vi "GUI - HDF (V1.00).vi"(0 "Time Data IN":refnum<class "GSwFormDSP.lvclass">, 5 "error in (no error)":errorcluster, 7 "Application Name":string="GSwForm", 9 "State Queue":string[](array[string])=["SC: Initialize"], 11 "HDF - READ":path, 13 "HDF - WRITE":path) -> (14 "Time Data DUP":refnum<class "GSwFormDSP.lvclass">, 19 "error out":errorcluster)   [LabVIEW 2020, in "HeadAcousticHDF.lvclass"]
uses:
  HeadAcousticHDF.lvclass
  API/GSwFormDSP_class/GSwFormDSP.lvclass
  <vilib>/Utility/sysdir.llb/System Directory Type.ctl
  C:/Users/fcharett/docsWork/coding/20openSourceSPWB/API/Generic Utilities_class/Generic Utilities.lvclass
  <vilib>/addons/_AddQ/G#Object/G#Object.lvclass
  API/Generic Utilities_class/Generic Utilities.lvclass
panel:
  in  "Task":enum32{"IO File", "File Info", "Settings"}(tab)
  out "Time Data":waveform(dbl)[](graph)
  in  "READ - Select HDF File":bool
  in  "WRITE - Select Wave File":bool
  in  "Select Channel":u16(ring)
  in  "File Info":bool
  out "State History":string[](array[string])
  out "State Index":i32
  in  "Exit":bool
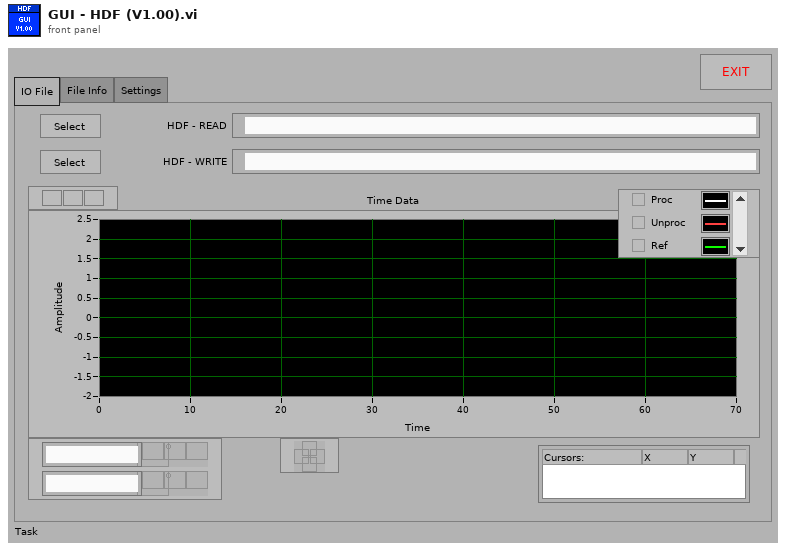
[diagram p1: front panel]
types:
  T1 = enum32{"Invalid", "Standard", "Closed", "Hidden", "Minimized", "Maximized"}
  T2 = typedef "System Directory Type.ctl" = i32
  T3 = cluster{"Name":string, "Unit":string, "Duration (sec)":dbl}[][]
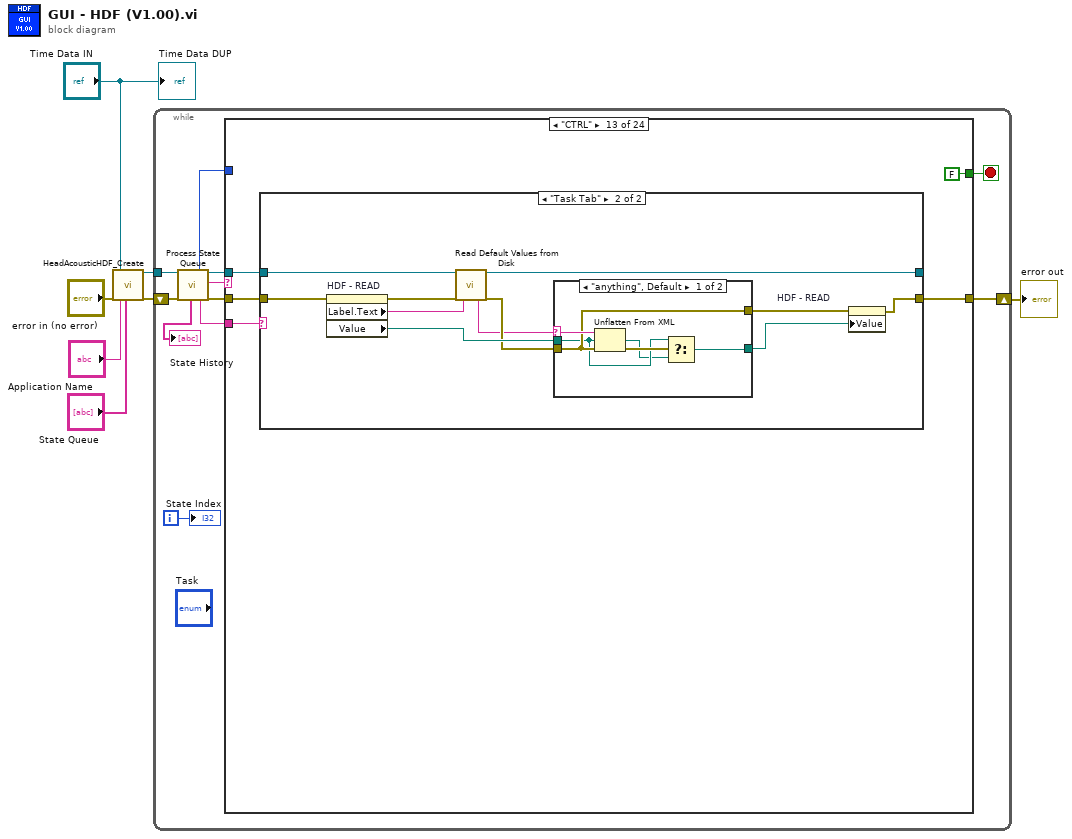
[diagram p0: block diagram]
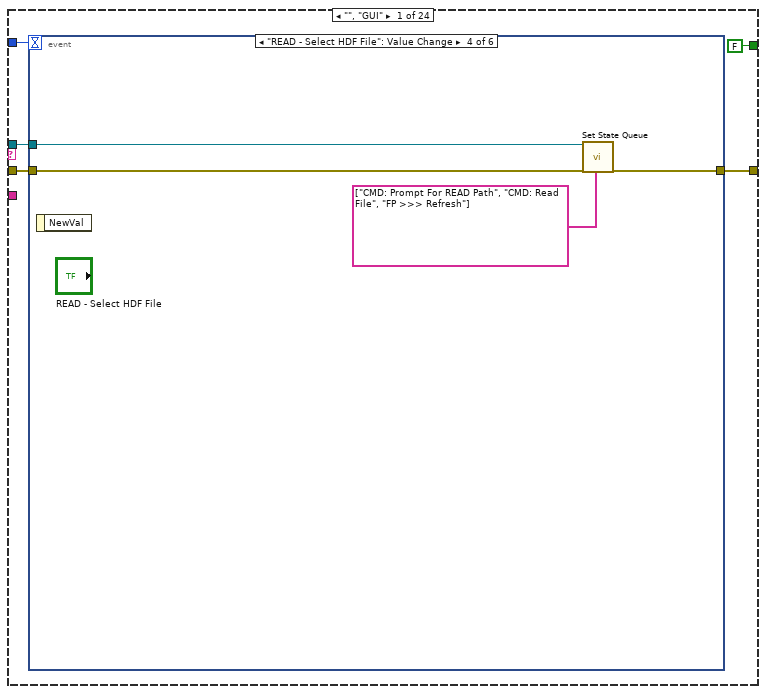
[diagram p2: hidden frame]
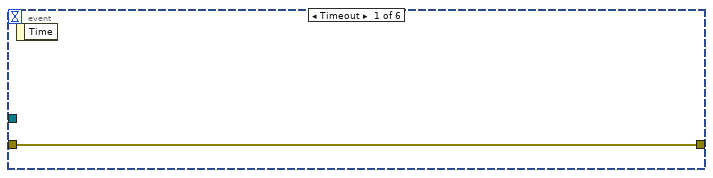
[diagram p3: hidden frame]
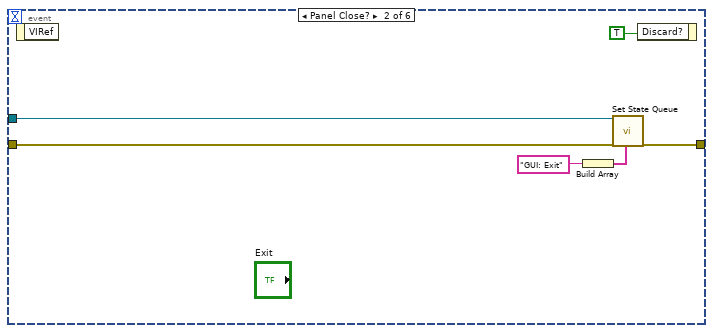
[diagram p4: hidden frame]
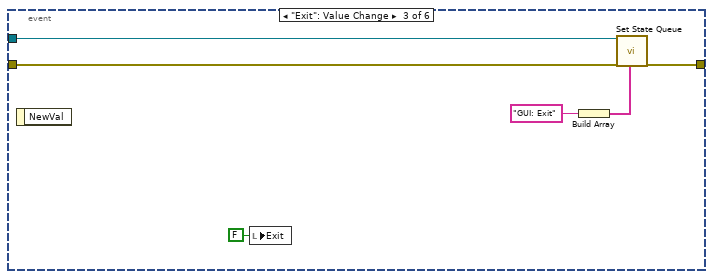
[diagram p5: hidden frame]
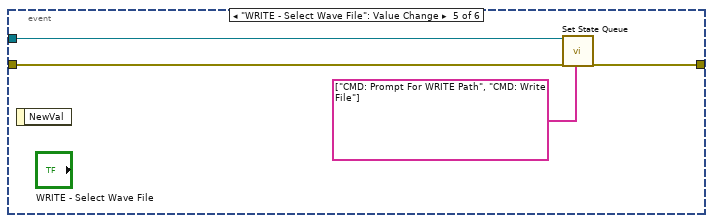
[diagram p6: hidden frame]
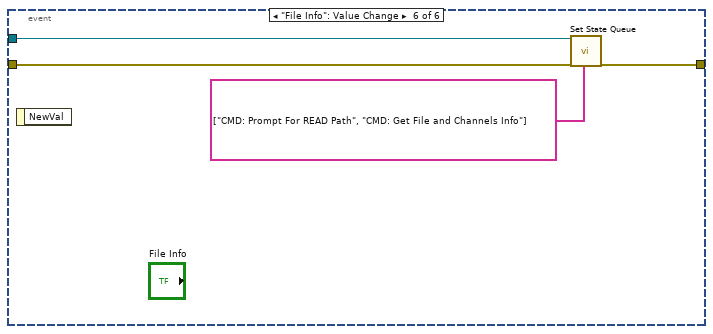
[diagram p7: hidden frame]
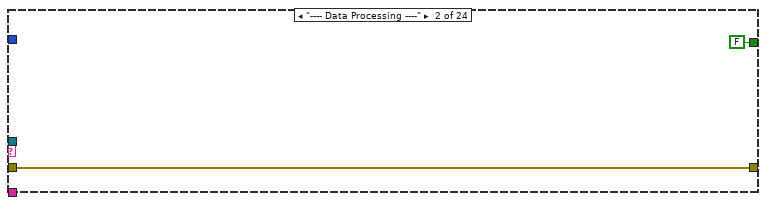
[diagram p8: hidden frame]
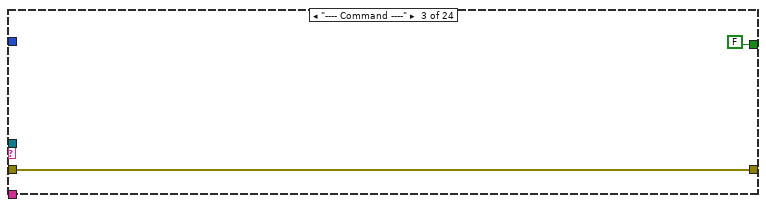
[diagram p9: hidden frame]
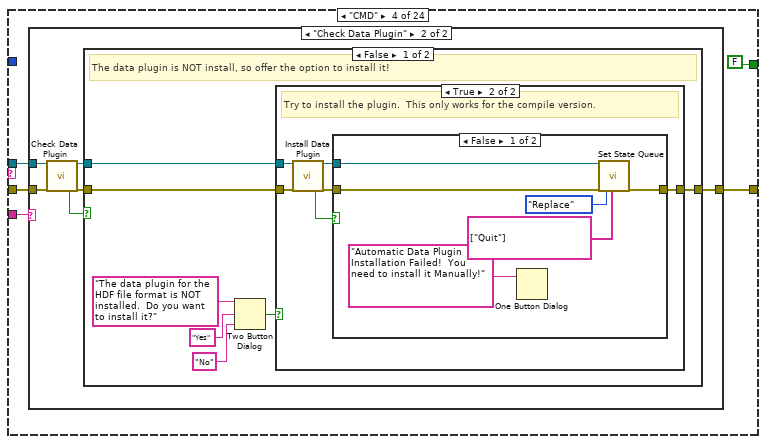
[diagram p10: hidden frame]
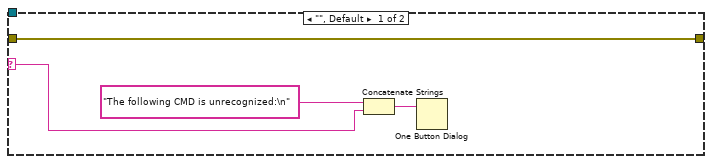
[diagram p11: hidden frame]
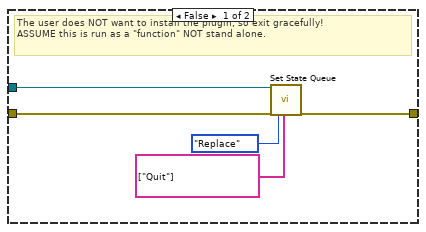
[diagram p12: hidden frame]
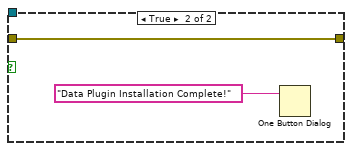
[diagram p13: hidden frame]
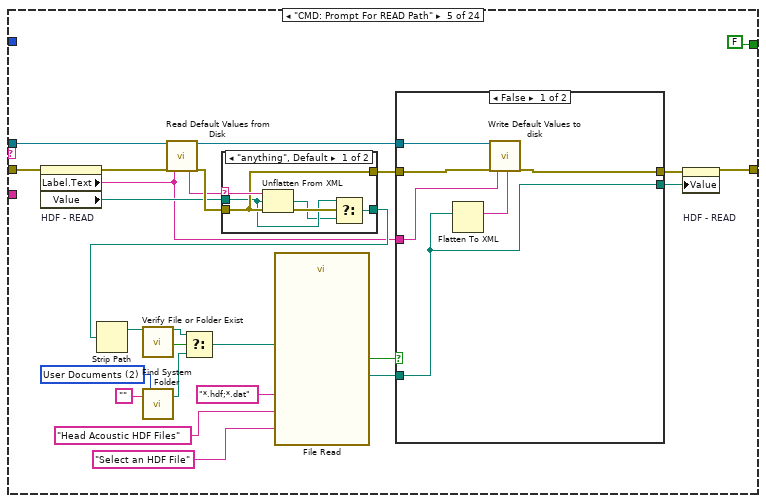
[diagram p15: hidden frame]
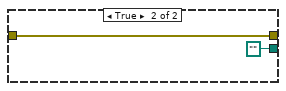
[diagram p16: hidden frame]
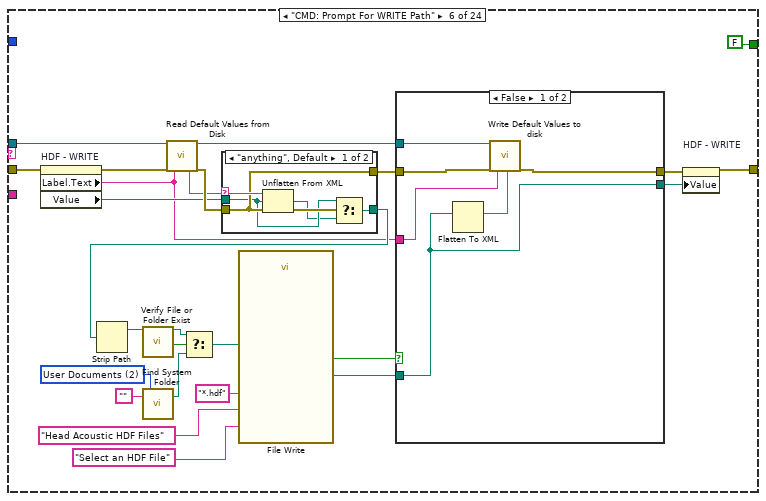
[diagram p18: hidden frame]
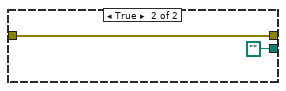
[diagram p19: hidden frame]
diagram:
  n1 = call "HeadAcousticHDF_Create.vi"("error in (no error)"="error in (no error)", "Time Data"="Time Data IN", "Application Name"="Application Name", "State Queue"="State Queue") -> ("reference out"=w7:refnum<class "HeadAcousticHDF.lvclass">, "error out"=w6:errorcluster)  [unwired: 14 in]
  n2 = while {
    shift-right: [w9] -> w2
    shift-left: w6 -> [w15]
    tunnel: w7 -> [w16]
    i -> [w17]
    stop <- w18 stop-if-true
    n3 = call "Process State Queue.vi"("reference in"=w16, "error in (no error)"=w15) -> ("State History"=→"State History":string[], "Timeout"=w14:i32, "State Option"=w11:string, "reference out"=w13:refnum<class "HeadAcousticHDF.lvclass">, "Current State"=w12:string, "error out"=w10:errorcluster)  [unwired: 10 in, 2 out]
    n4 = case shown="\"CTRL\"" w12 {
      selector: w12 -> [_ _ _ _ _ _ _ _ _ _ _ _ _ _ _ _ _ _ _ _ w403 _ _ _]
      tunnel: w13 -> [w21 _ _ w53 w119 w161 w183 w195 w208 _ w231 _ w237 w267 _ w308 w327 w360 w385 _ _ _ _ w411]
      tunnel: [FALSE FALSE FALSE FALSE FALSE FALSE FALSE FALSE FALSE FALSE FALSE FALSE FALSE FALSE FALSE FALSE TRUE FALSE FALSE FALSE FALSE FALSE FALSE TRUE] -> w18
      tunnel: w14 -> [w22 _ _ _ _ _ _ _ _ _ _ _ _ _ _ _ _ _ _ _ _ _ _ _]
      tunnel: w11 -> [_ _ _ w56 _ _ _ _ _ _ _ _ w238 w264 _ _ _ w369 _ _ _ _ _ _]
      tunnel: w10 -> [w20 w49 w51 w54 w118 w160 w182 w194 w209 w226 w230 w233 w235 w266 w293 w305 w324 w359 w386 w399 w401 w406 w409 w412]
      tunnel: [w19 w49 w51 w55 w102 w146 w181 w193 w204 w226 w229 w233 w236 w265 w293 w295 w323 w357 w382 w399 w401 errorcluster {"status"=FALSE, "code"=0, "source"=""} ("error out") w409 w413] -> w9
      frame "", "GUI" {
        n5 = event shown="[3] \"READ - Select HDF File\": Value Change" {
          selector: _ -> [_ _ _ _ _ _]
          dyn-events: _ -> [_ _ _ _ _ _]
          timeout: w22 -> [_ _ _ _ _ _]
          tunnel: w21 -> [_ w28 w34 w39 w43 w45]
          tunnel: w20 -> [w24 w27 w32 w38 w42 w46]
          tunnel: [w24 w26 w33 w40 w44 w47] -> w19
          event Timeout {
            n6 = event-data() -> ()  [unwired: 1 in, 1 out]
          }
          event Panel Close? {
            n7 = event-data() -> ()  [unwired: 1 in, 1 out]
            n8 = Build Array("GUI: Exit") -> (w25:string[])
            n9 = call "Set State Queue.vi"("reference in"=w28, "error in (no error)"=w27, "State Queue"=w25) -> ("error out"=w26:errorcluster)  [unwired: 15 in, 1 out]
            n10 = event-data("Discard?"=TRUE) -> ()  [unwired: 1 in, 1 out]
          }
          event "Exit": Value Change {
            n11 = event-data() -> ()  [unwired: 1 in, 1 out]
            n12 = local write "Exit"(FALSE ("Exit")) -> ()
            n13 = Build Array("GUI: Exit") -> (w31:string[])
            n14 = call "Set State Queue.vi"("reference in"=w34, "error in (no error)"=w32, "State Queue"=w31) -> ("error out"=w33:errorcluster)  [unwired: 15 in, 1 out]
          }
          event "READ - Select HDF File": Value Change {
            n15 = event-data() -> ()  [unwired: 1 in, 1 out]
            n16 = call "Set State Queue.vi"("reference in"=w39, "error in (no error)"=w38, "State Queue"=string[] ["CMD: Prompt For READ Path", "CMD: Read File", "FP >>> Refresh"]) -> ("error out"=w40:errorcluster)  [unwired: 15 in, 1 out]
          }
          event "WRITE - Select Wave File": Value Change {
            n17 = event-data() -> ()  [unwired: 1 in, 1 out]
            n18 = call "Set State Queue.vi"("reference in"=w43, "error in (no error)"=w42, "State Queue"=string[] ["CMD: Prompt For WRITE Path", "CMD: Write File"]) -> ("error out"=w44:errorcluster)  [unwired: 15 in, 1 out]
          }
          event "File Info": Value Change {
            n19 = event-data() -> ()  [unwired: 1 in, 1 out]
            n20 = call "Set State Queue.vi"("reference in"=w45, "error in (no error)"=w46, "State Queue"=string[] ["CMD: Prompt For READ Path", "CMD: Get File and Channels Info"]) -> ("error out"=w47:errorcluster)  [unwired: 15 in, 1 out]
          }
        }
      }
      frame "---- Data Processing ----" {
      }
      frame "---- Command ----" {
      }
      frame "CMD" {
        n21 = case shown="\"Check Data Plugin\"" w56 {
          selector: w56 -> [w59 _]
          tunnel: [w58 w64] -> w55
          tunnel: w54 -> [w58 w66]
          tunnel: w53 -> [_ w67]
          frame "", Default {
            n22 = Concatenate Strings("The following CMD is unrecognized:\n", w59) -> (w60:string)
            n23 = One Button Dialog(message=w60) -> ()  [unwired: 1 in, 1 out]
          }
          frame "Check Data Plugin" {
            n24 = call "Check Data Plugin.vi"("reference in"=w67, "error in (no error)"=w66) -> ("HDF Plugin OK?"=w65:bool, "reference out"=w62:refnum<class "HeadAcousticHDF.lvclass">, "error out"=w63:errorcluster)  [unwired: 15 in]
            n25 = case shown="False" w65 {
              tunnel: [w69 w94] -> w64
              tunnel: w63 -> [w70 w94]
              tunnel: w62 -> [w71 _]
              frame False {
                # "The data plugin is NOT install, so offer the option to install it!"
                n26 = Two Button Dialog(message="The data plugin for the HDF file format is NOT installed.  Do you want to install it?", 1:"No" ("F button name (\"Cancel\")"), 2:"Yes" ("T button name (\"OK\")")) -> (T button?=w72:bool)
                n27 = case shown="True" w72 {
                  tunnel: w71 -> [w79 w85]
                  tunnel: w70 -> [w78 w84]
                  tunnel: [w77 w82] -> w69
                  frame False {
                    # "The user does NOT want to install the plugin, so exit gracefully!\nASSUME this is run as a \"function\" NOT stand alone."
                    n28 = call "Set State Queue.vi"("reference in"=w79, "error in (no error)"=w78, "State Queue Options"=enum16{"Replace", "Append", "Prepend"}."Replace", "State Queue"=string[] ["Quit"]) -> ("error out"=w77:errorcluster)  [unwired: 14 in, 1 out]
                  }
                  frame True {
                    # "Try to install the plugin.  This only works for the compile version."
                    n29 = call "Install Data Plugin.vi"("reference in"=w85, "error in (no error)"=w84) -> ("Successful Install?"=w83:bool, "reference out"=w80:refnum<class "HeadAcousticHDF.lvclass">, "error out"=w81:errorcluster)  [unwired: 15 in]
                    n30 = case shown="False" w83 {
                      tunnel: [w86 w92] -> w82
                      tunnel: w81 -> [w87 w92]
                      tunnel: w80 -> [w88 _]
                      frame False {
                        n31 = One Button Dialog(message="Automatic Data Plugin Installation Failed!  You need to install it Manually!") -> ()  [unwired: 1 in, 1 out]
                        n32 = call "Set State Queue.vi"("reference in"=w88, "error in (no error)"=w87, "State Queue Options"=enum16{"Replace", "Append", "Prepend"}."Replace", "State Queue"=string[] ["Quit"]) -> ("error out"=w86:errorcluster)  [unwired: 14 in, 1 out]
                      }
                      frame True {
                        n33 = One Button Dialog(message="Data Plugin Installation Complete!") -> ()  [unwired: 1 in, 1 out]
                      }
                    }
                  }
                }
              }
              frame True {
                # "The data plugin is OK"
              }
            }
          }
        }
      }
      frame "CMD: Prompt For READ Path" {
        w109 = T2 2 items=["User Home"=0, "User Desktop"=1, "User Documents"=2, "User Application Data"=3, "User Preferences"=4, "User Temporary"=5, "Public Documents"=6, "Public Application Data"=7, "Public Preferences"=8, "Public Cache"=13, "System Core Libraries"=9, "System Installed Libraries"=10, "Application Files"=11, "Boot Volume Root"=12] ("system directory type")
        n34 = property on="HDF - READ" class="Path"(error in=w118) -> (error out=w117:errorcluster, "Label.Text"=w97:string, "Value"=w115:path)  [unwired: 1 in, 1 out]
        n35 = call "Find System Folder.vi"("Application Name"="", "system directory type"=w109) -> ("System Folder"=w108:path)  [unwired: 16 in, 1 out]
        n36 = call-dynamic "Read Default Values from Disk.vi"("reference in"=w119, "error in (no error)"=w117, "Control Label"=w97) -> ("Value (XML String)"=w95:string, "reference out"=w98:refnum<class "HeadAcousticHDF.lvclass">, "error out"=w116:errorcluster)  [unwired: 14 in]
        n37 = case shown="\"anything\", Default" w95 {
          selector: w95 -> [w134 _]
          tunnel: [w129 w136] -> w114
          tunnel: w115 -> [w131 w136]
          tunnel: w116 -> [w132 w135]
          tunnel: [w132 w135] -> w100
          frame "anything", Default {
            n38 = Unflatten From XML(xml string=w134, type=w131, error in (no error)=w132) -> (value=w130:path, error out=w133:errorcluster)
            n39 = Select(t=w131, s=w133, f=w130) -> (s? t:f=w129:path)
          }
          frame "" {
            # "Either the file was not found or there was some error"
          }
        }
        n40 = Strip Path(path=w114) -> (stripped path=w113:path)  [unwired: 1 out]
        n41 = call "Verify File or Folder Exist.vi"("path"=w113) -> ("dup path"=w111:path, "file or folder exists?"=w112:bool)  [unwired: 16 in, 1 out]
        n42 = Select(t=w111, s=w112, f=w108) -> (s? t:f=w110:path)
        n43 = call "File Read"("start path"=w110, "button label"="Select an HDF File", "pattern (all files)"="*.hdf;*.dat", "pattern label"="Head Acoustic HDF Files") -> ("selected path"=w96:path, "cancelled"=w103:bool)  [unwired: 8 in, 2 out]
        n44 = case shown="False" w103 {
          tunnel: [w122 w128] -> w101
          tunnel: w100 -> [w123 w128]
          tunnel: [w121 path ""] -> w99
          tunnel: w98 -> [w125 _]
          tunnel: w97 -> [w124 _]
          tunnel: w96 -> [w121 _]
          frame False {
            n45 = Flatten To XML(6:w121) -> (2:w126:string)
            n46 = call-dynamic "Write Default Values to disk.vi"("reference in"=w125, "error in (no error)"=w123, "Control Label"=w124, "Value (XML String)"=w126) -> ("error out"=w122:errorcluster)  [unwired: 14 in, 1 out]
          }
          frame True {
          }
        }
        n47 = property on="HDF - READ" class="Path"(error in=w101, "Value"=w99) -> (error out=w102:errorcluster)  [unwired: 1 in, 1 out]
      }
      frame "CMD: Prompt For WRITE Path" {
        w151 = T2 2 items=["User Home"=0, "User Desktop"=1, "User Documents"=2, "User Application Data"=3, "User Preferences"=4, "User Temporary"=5, "Public Documents"=6, "Public Application Data"=7, "Public Preferences"=8, "Public Cache"=13, "System Core Libraries"=9, "System Installed Libraries"=10, "Application Files"=11, "Boot Volume Root"=12] ("system directory type")
        n48 = property on="HDF - WRITE" class="Path"(error in=w160) -> (error out=w159:errorcluster, "Label.Text"=w141:string, "Value"=w157:path)  [unwired: 1 in, 1 out]
        n49 = call "Find System Folder.vi"("Application Name"="", "system directory type"=w151) -> ("System Folder"=w150:path)  [unwired: 16 in, 1 out]
        n50 = call-dynamic "Read Default Values from Disk.vi"("reference in"=w161, "error in (no error)"=w159, "Control Label"=w141) -> ("Value (XML String)"=w137:string, "reference out"=w142:refnum<class "HeadAcousticHDF.lvclass">, "error out"=w158:errorcluster)  [unwired: 14 in]
        n51 = case shown="\"anything\", Default" w137 {
          selector: w137 -> [w176 _]
          tunnel: [w171 w178] -> w156
          tunnel: w157 -> [w173 w178]
          tunnel: w158 -> [w174 w177]
          tunnel: [w174 w177] -> w144
          frame "anything", Default {
            n52 = Unflatten From XML(xml string=w176, type=w173, error in (no error)=w174) -> (value=w172:path, error out=w175:errorcluster)
            n53 = Select(t=w173, s=w175, f=w172) -> (s? t:f=w171:path)
          }
          frame "" {
            # "Either the file was not found or there was some error"
          }
        }
        n54 = Strip Path(path=w156) -> (stripped path=w155:path)  [unwired: 1 out]
        n55 = call "Verify File or Folder Exist.vi"("path"=w155) -> ("dup path"=w153:path, "file or folder exists?"=w154:bool)  [unwired: 16 in, 1 out]
        n56 = Select(t=w153, s=w154, f=w150) -> (s? t:f=w152:path)
        n57 = call "File Write"("start path"=w152, "button label"="Select an HDF File", "pattern (all files)"="*.hdf", "pattern label"="Head Acoustic HDF Files") -> ("selected path"=w140:path, "cancelled"=w147:bool)  [unwired: 8 in, 2 out]
        n58 = case shown="False" w147 {
          tunnel: [w164 w170] -> w145
          tunnel: w144 -> [w165 w170]
          tunnel: [w163 path ""] -> w143
          tunnel: w142 -> [w167 _]
          tunnel: w141 -> [w166 _]
          tunnel: w140 -> [w163 _]
          frame False {
            n59 = Flatten To XML(6:w163) -> (2:w168:string)
            n60 = call-dynamic "Write Default Values to disk.vi"("reference in"=w167, "error in (no error)"=w165, "Control Label"=w166, "Value (XML String)"=w168) -> ("error out"=w164:errorcluster)  [unwired: 14 in, 1 out]
          }
          frame True {
          }
        }
        n61 = property on="HDF - WRITE" class="Path"(error in=w145, "Value"=w143) -> (error out=w146:errorcluster)  [unwired: 1 in, 1 out]
      }
      frame "CMD: Read File" {
        n62 = Empty String/Path?(string/path="HDF - READ") -> (empty?=w180:bool)
        n63 = case shown="False" w180 {
          tunnel: w183 -> [w185 _]
          tunnel: w182 -> [w186 w190]
          tunnel: [w188 w190] -> w181
          tunnel: "HDF - READ" -> [w187 _]
          frame False {
            n64 = call "READ - File.vi"("reference in"=w185, "error in (no error)"=w186, "Path - READ"=w187, "Channel Selected (0=ALL)"="Select Channel") -> ("error out"=w188:errorcluster)  [unwired: 14 in, 1 out]
          }
          frame True {
            # "User cancelled, so do nothing!"
          }
        }
      }
      frame "CMD: Write File" {
        n65 = Empty String/Path?(string/path="HDF - WRITE") -> (empty?=w192:bool)
        n66 = case shown="False" w192 {
          tunnel: w195 -> [w198 _]
          tunnel: w194 -> [w197 w201]
          tunnel: [w200 w201] -> w193
          tunnel: "HDF - WRITE" -> [w199 _]
          frame False {
            n67 = call "WRITE - File.vi"("reference in"=w198, "error in (no error)"=w197, "TDMS Path - WRITE"=w199) -> ("error out"=w200:errorcluster)  [unwired: 15 in, 1 out]
          }
          frame True {
            # "User cancelled, so do nothing!"
          }
        }
      }
      frame "CMD: Get File and Channels Info" {
        n68 = local read "HDF - READ"() -> (w206:path)
        n69 = Empty String/Path?(string/path=w206) -> (empty?=w207:bool)
        n70 = case shown="False" w207 {
          tunnel: w209 -> [w217 w225]
          tunnel: w208 -> [w216 _]
          tunnel: w206 -> [w215 _]
          tunnel: [w214 w225] -> w205
          tunnel: [w211 string[] []] -> w203
          frame False {
            n71 = call "READ - File & Channels INFO.vi"("reference in"=w216, "error in (no error)"=w217, "Path - READ"=w215) -> ("Channel info"=w213:T3, "error out"=w214:errorcluster)  [unwired: 14 in, 1 out]
            n72 = for {
              tunnel: w213 -> [w221] mode=indexing
              shift-right: [w219] -> w211
              shift-left: string[] ["All"] -> [w218]
              n73 = for {
                tunnel: w221 -> [w223] mode=indexing
                tunnel: [w222] -> w220 mode=indexing
                n74 = Unbundle By Name(w223) -> ("Name"=w222:string)
              }
              n75 = Build Array (concatenate)(w218, w220) -> (w219:string[])
            }
          }
          frame True {
          }
        }
        n76 = property on="Select Channel" class="Ring (strict)"(error in=w205, "Strings []"=w203, "Value"=0) -> (error out=w204:errorcluster)  [unwired: 1 in, 1 out]
      }
      frame "---- Scripts ----" {
      }
      frame "SC: Initialize" {
        n77 = call "Set State Queue.vi"("reference in"=w231, "error in (no error)"=w230, "State Queue"=string[] ["GUI: Initialize Ref", "CMD >>> Check Data Plugin", "FP >>> Open"] ("State Queue OUT")) -> ("error out"=w229:errorcluster)  [unwired: 15 in, 1 out]
      }
      frame "---- Front Panel Mgmt ----" {
      }
      frame "CTRL" {
        n78 = case shown="\"Task Tab\"" w238 {
          selector: w238 -> [w243 _]
          tunnel: [w241 w248] -> _
          tunnel: w237 -> [w241 w253]
          tunnel: [w240 w247] -> w236
          tunnel: w235 -> [w240 w251]
          frame "unknown", Default {
            n79 = Concatenate Strings("The following control name is unrecognized:\n", w243) -> (w242:string)
            n80 = One Button Dialog(message=w242) -> ()  [unwired: 1 in, 1 out]
          }
          frame "Task Tab" {
            n81 = property on="HDF - READ" class="Path"(error in=w251) -> (error out=w252:errorcluster, "Label.Text"=w250:string, "Value"=w255:path)  [unwired: 1 in, 1 out]
            n82 = call-dynamic "Read Default Values from Disk.vi"("reference in"=w253, "error in (no error)"=w252, "Control Label"=w250) -> ("Value (XML String)"=w245:string, "reference out"=w248:refnum<class "HeadAcousticHDF.lvclass">, "error out"=w249:errorcluster)  [unwired: 14 in]
            n83 = case shown="\"anything\", Default" w245 {
              selector: w245 -> [w261 _]
              tunnel: [w256 w263] -> w246
              tunnel: w255 -> [w258 w263]
              tunnel: w249 -> [w259 w262]
              tunnel: [w259 w262] -> w254
              frame "anything", Default {
                n84 = Unflatten From XML(xml string=w261, type=w258, error in (no error)=w259) -> (value=w257:path, error out=w260:errorcluster)
                n85 = Select(t=w258, s=w260, f=w257) -> (s? t:f=w256:path)
              }
              frame "" {
                # "Either the file was not found or there was some error"
              }
            }
            n86 = property on="HDF - READ" class="Path"(error in=w254, "Value"=w246) -> (error out=w247:errorcluster)  [unwired: 1 in, 1 out]
          }
        }
      }
      frame "FP" {
        n87 = case shown="\"Refresh\"" w264 {
          selector: w264 -> [w269 _ _]
          tunnel: w267 -> [_ w277 w290]
          tunnel: w266 -> [w270 w276 w289]
          tunnel: [w270 w273 w287] -> w265
          frame "", Default {
            n88 = Concatenate Strings("The following FP is unrecognized:\n", w269) -> (w271:string)
            n89 = One Button Dialog(message=w271) -> ()  [unwired: 1 in, 1 out]
          }
          frame "Open" {
            n90 = call-dynamic "Get VI Ref.vi"("reference in"=w277, "error in (no error)"=w276) -> ("GUI VI Ref"=w274:refnum<vi>, "error out"=w275:errorcluster)  [unwired: 14 in, 2 out]
            n91 = property class="VI"(reference=w274, error in=w275) -> (reference out=w279:refnum<vi>, error out=w280:errorcluster, "Front Panel.Open"=w278:bool)
            n92 = case shown="False" w278 {
              tunnel: [w283 w286] -> w273
              tunnel: w280 -> [w282 w286]
              tunnel: w279 -> [w281 _]
              frame False {
                n93 = invoke class="VI" method="FP.Open"(reference=w281, error in=w282, "Activate"=TRUE, "State"=T1."Standard") -> (error out=w283:errorcluster)  [unwired: 1 in, 4 out]
              }
              frame True {
              }
            }
          }
          frame "Refresh" {
            n94 = call "Get - Time Data OBJ.vi"("reference in"=w290, "error in (no error)"=w289) -> ("Time Data OBJ"=w292:refnum<class "GSwFormDSP.lvclass">, "error out"=w291:errorcluster)  [unwired: 15 in, 1 out]
            n95 = call-dynamic "Get - wForms.vi"("reference in"=w292, "error in (no error)"=w291) -> ("wForms"=→"Time Data":waveform(dbl)[], "error out"=w287:errorcluster)  [unwired: 14 in, 2 out]
          }
        }
      }
      frame "---- GUI Functions ----" {
      }
      frame "GUI: Initialize Ref" {
        n96 = control-ref of="GUI Reference"() -> (w304:refnum<vi>)
        n97 = call "Set VI Ref.vi"("reference in"=w308, "error in (no error)"=w305, "ReInit All to Default?"=FALSE, "GUI VI Ref"=w304) -> ("reference out"=w307:refnum<class "HeadAcousticHDF.lvclass">, "error out"=w303:errorcluster)  [unwired: 14 in]
        n98 = call "Set Close Panel (Yes or No).vi"("reference in"=w307, "error in (no error)"=w303) -> ("reference out"=w306:refnum<class "HeadAcousticHDF.lvclass">, "error out"=w302:errorcluster)  [unwired: 16 in]
        n99 = call "Set Message Window Ref.vi"("reference in"=w306, "error in (no error)"=w302) -> ("reference out"=w300:refnum<class "HeadAcousticHDF.lvclass">, "error out"=w299:errorcluster)  [unwired: 16 in]
        n100 = call "Get - Time Data OBJ State.vi"("reference in"=w300, "error in (no error)"=w299) -> ("New Time Data Obj?"=w296:bool, "reference out"=w298:refnum<class "HeadAcousticHDF.lvclass">, "error out"=w297:errorcluster)  [unwired: 15 in]
        n101 = case shown="True" w296 {
          tunnel: w298 -> [_ w316]
          tunnel: w297 -> [w310 w315]
          tunnel: [w310 w311] -> w295
          frame False {
          }
          frame True {
            n102 = call "Get - Time Data OBJ.vi"("reference in"=w316, "error in (no error)"=w315) -> ("Time Data OBJ"=w313:refnum<class "GSwFormDSP.lvclass">, "error out"=w312:errorcluster)  [unwired: 15 in, 1 out]
            n103 = call "Set - wForms.vi"("reference in"=w313, "error in (no error)"=w312, "Init wForms"=TRUE) -> ("error out"=w311:errorcluster)  [unwired: 15 in, 1 out]
          }
        }
      }
      frame "GUI: Exit" {
        n104 = call-dynamic "Get Message Window Ref.vi"("reference in"=w327, "error in (no error)"=w324) -> ("reference out"=w326:refnum<class "HeadAcousticHDF.lvclass">, "Msg Win Ref"=w322:refnum<vi>, "error out"=w325:errorcluster)  [unwired: 15 in]
        n105 = call-dynamic "Get VI Ref.vi"("reference in"=w326, "error in (no error)"=w325) -> ("reference out"=w331:refnum<class "HeadAcousticHDF.lvclass">, "GUI VI Ref"=w329:refnum<vi>, "error out"=w330:errorcluster)  [unwired: 14 in, 1 out]
        n106 = call-dynamic "Get Close Panel (Yes or No).vi"("reference in"=w331, "error in (no error)"=w330) -> ("Close Panel?"=w332:bool, "reference out"=w321:refnum<class "HeadAcousticHDF.lvclass">, "error out"=w319:errorcluster)  [unwired: 15 in]
        n107 = call "Get - Time Data OBJ State.vi"("reference in"=w321, "error in (no error)"=w319) -> ("New Time Data Obj?"=w317:bool, "reference out"=w320:refnum<class "HeadAcousticHDF.lvclass">, "error out"=w318:errorcluster)  [unwired: 15 in]
        n108 = call-dynamic "Destroy.vi"("reference in"=w320, "error in (no error)"=w318) -> ("error out"=w336:errorcluster)  [unwired: 16 in, 1 out]
        n109 = case shown="True" w317 {
          tunnel: w336 -> [w338 w340]
          tunnel: [w338 w339] -> w328
          frame False {
          }
          frame True {
            n110 = call <vilib>:"GarbageCollector.vi"("error in (no error)"=w340) -> ("error out"=w339:errorcluster)  [unwired: 16 in, 2 out]
          }
        }
        n111 = Close Reference(reference=w322, error in (no error)=w328) -> (error out=w335:errorcluster)
        n112 = case shown="True" w332 {
          tunnel: w335 -> [w342 w346]
          tunnel: [w342 w345] -> w333
          tunnel: [w341 w344] -> w334
          tunnel: w329 -> [w341 w343]
          frame False {
          }
          frame True {
            n113 = property class="VI"(reference=w343, error in=w346) -> (reference out=w348:refnum<vi>, error out=w347:errorcluster, "Front Panel.Open"=w349:bool)
            n114 = case shown="True" w349 {
              tunnel: [w351 w355] -> w345
              tunnel: w347 -> [w351 w354]
              tunnel: w348 -> [w350 w353]
              tunnel: [w350 w352] -> w344
              frame False {
              }
              frame True {
                n115 = invoke class="VI" method="FP.Close"(reference=w353, error in=w354) -> (reference out=w352:refnum<vi>, error out=w355:errorcluster)  [unwired: 1 in, 1 out]
              }
            }
          }
        }
        n116 = Close Reference(reference=w334, error in (no error)=w333) -> (error out=w323:errorcluster)
      }
      frame "SEND MSG" {
        n117 = call-dynamic "Get Message Window Ref.vi"("reference in"=w360, "error in (no error)"=w359) -> ("Msg Win Ref"=w356:refnum<vi>, "error out"=w358:errorcluster)  [unwired: 15 in, 1 out]
        n118 = property class="VI"(reference=w356, error in=w358) -> (reference out=w362:refnum<vi>, error out=w361:errorcluster, "Front Panel.Open"=w363:bool)
        n119 = case shown="False" w363 {
          tunnel: [w377 w381] -> w365
          tunnel: w361 -> [w372 w381]
          tunnel: w362 -> [w374 w380]
          tunnel: [w376 w380] -> w364
          frame False {
            w375 = FALSE ("Wait Until Done")
            n120 = invoke class="VI" method="Run VI"(reference=w374, error in=w372, "Wait until done"=w375, "Auto Dispose Ref"=w375) -> (reference out=w373:refnum<vi>, error out=w371:errorcluster)  [unwired: 1 in, 3 out]
            n121 = invoke class="VI" method="FP.Open"(reference=w373, error in=w371, "Activate"=TRUE, "State"=T1."Standard") -> (reference out=w376:refnum<vi>, error out=w377:errorcluster)  [unwired: 1 in, 3 out]
          }
          frame True {
          }
        }
        n122 = Concatenate Strings("\r\n", w369) -> (w368:string)
        n123 = invoke class="VI" method="Ctrl Val.Set"(reference=w364, error in=w365, "Control Name"="Message", "Value"=w368) -> (error out=w357:errorcluster)  [unwired: 1 in, 4 out]
      }
      frame "CLOSE MSG" {
        n124 = call-dynamic "Get Message Window Ref.vi"("reference in"=w385, "error in (no error)"=w386) -> ("Msg Win Ref"=w383:refnum<vi>, "error out"=w384:errorcluster)  [unwired: 15 in, 1 out]
        n125 = property class="VI"(reference=w383, error in=w384) -> (reference out=w390:refnum<vi>, error out=w391:errorcluster, "Front Panel.Open"=w389:bool)
        n126 = case shown="True" w389 {
          tunnel: [w394 w398] -> w388
          tunnel: w391 -> [w394 w397]
          tunnel: w390 -> [w393 w396]
          tunnel: [w393 w395] -> w387
          frame False {
          }
          frame True {
            n127 = invoke class="VI" method="FP.Close"(reference=w396, error in=w397) -> (reference out=w395:refnum<vi>, error out=w398:errorcluster)  [unwired: 1 in, 1 out]
          }
        }
        n128 = invoke class="VI" method="Abort VI"(reference=w387, error in=w388) -> (error out=w382:errorcluster)  [unwired: 1 in, 2 out]
      }
      frame "---- Miscelleneous ----" {
      }
      frame "unknown", Default {
        n129 = Concatenate Strings("The following state is unrecognized?\n", w403) -> (w402:string)
        n130 = One Button Dialog(message=w402) -> ()  [unwired: 1 in, 1 out]
      }
      frame "Error" {
        n131 = call <vilib>:"General Error Handler.vi"("error in (no error)"=w406) -> ()  [unwired: 10 in, 5 out]
      }
      frame "Next" {
        # "This is an empty case used so the queue does NOT stop if there is an empty string between two valid states!"
      }
      frame "Quit" {
        # "This is the case used to simply exit when this GUI is used as a SubVI!"
        n132 = call-dynamic "Destroy.vi"("reference in"=w411, "error in (no error)"=w412) -> ("error out"=w413:errorcluster)  [unwired: 16 in, 1 out]
      }
    }
    "State Index" <- w17
  }
  "error out" <- w2
  "Time Data DUP" <- "Time Data IN"
